vi "RSZVB Set Virtual Transform Ground Loop State.vi"(7 "State (Off)":bool, 8 "error in (no error)":errorcluster {"code" format="%.0x"}, 9 "Function Type (0)":i32(ring) items=["Deembedding", "Embedding"], 10 "Channel (1)":i32=1, 11 "VISA session":refnum<visa-resource-name>) -> (0 "error out":errorcluster {"code" format="%.0x"}, 3 "dup VISA session":refnum<visa-resource-name>)   [LabVIEW 2011]
doc: "This VI enables or disables the deembedding/embedding VI for ground loops. It is allowed to change the circuit model and its parameters while deembedding is enabled.\n\nRemote-control command(s):\nCALCulate<Ch>:TRANsform:VNETworks:GLOop:DEEMbedding[:STATe] ON | OFF\nCALCulate<Ch>:TRANsform:VNETworks:GLOop:EMBedding[:STATe] ON | OFF"
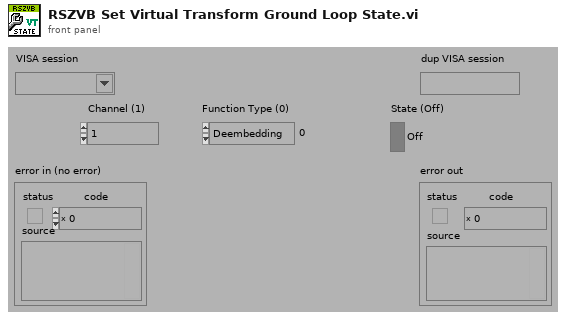
[diagram p1: front panel]
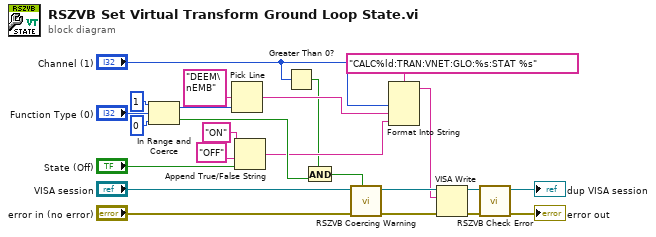
[diagram p0: block diagram]
diagram:
  n1 = In Range and Coerce(upper limit=1, x="Function Type (0)", lower limit=0) -> (coerced(x)=w15:i32, In Range?=w11:bool)
  n2 = Pick Line(multi-line string="DEEM\nEMB", line index=w15) -> (output string=w6:string)  [unwired: 1 in]
  n3 = Append True/False String(1:"State (Off)", 2:"OFF" ("false string"), 3:"ON" ("true string")) -> (0:w8:string)  [unwired: 1 in]
  n4 = Greater Than 0?(x="Channel (1)") -> (x > 0?=w5:bool)
  n5 = And(x=w5, y=w11) -> (x .and. y?=w3:bool)
  n6 = call "RSZVB Coercing Warning.vi"("In Range?"=w3, "error in (no error)"="error in (no error)", "VISA session"="VISA session") -> ("error out"=w18:errorcluster, "dup VISA session"=w19:refnum<visa-resource-name>)  [unwired: 7 in]
  n7 = Format Into String(format string="CALC%ld:TRAN:VNET:GLO:%s:STAT %s", "Channel (1)", w6, w8) -> (resulting string=w17:string)  [unwired: 2 in, 1 out]
  n8 = VISA Write(VISA resource name=w19, write buffer=w17, error in (no error)=w18) -> (VISA resource name out=w22:refnum<visa-resource-name>, error out=w21:errorcluster)  [unwired: 1 out]
  n9 = call "RSZVB Check Error.vi"("error in (no error)"=w21, "VISA session"=w22) -> ("error out"=→"error out":errorcluster, "dup VISA session"=→"dup VISA session":refnum<visa-resource-name>)  [unwired: 8 in]
